vi "Path_2_String.vi"(1 "Real Path":path) -> (0 "Path String":string)   [LabVIEW 2022 SP3]
uses:
  Globals/Constants_global.vi
  Globals/Preference_global.vi
panel:
  in  "POSIXFormattedPseudopath (F)":bool
  out "Data Folder":path
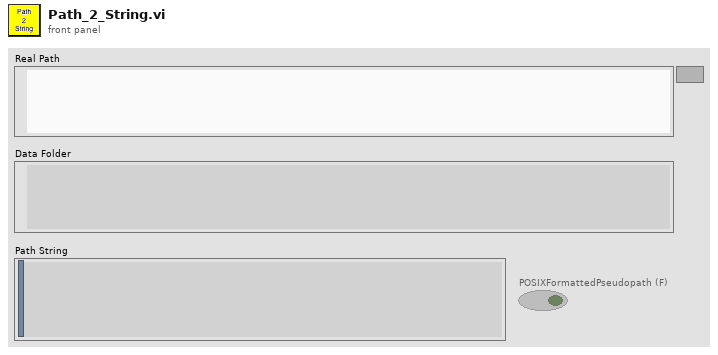
[diagram p1: front panel]
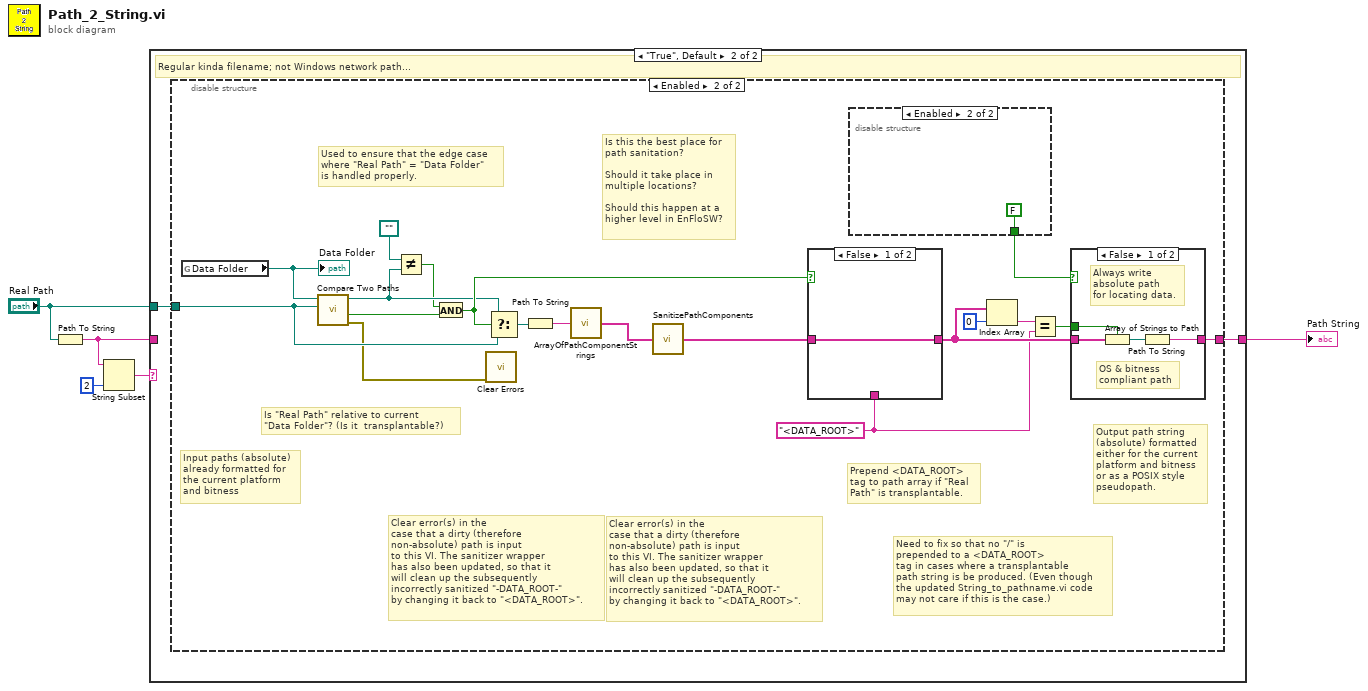
[diagram p0: block diagram]
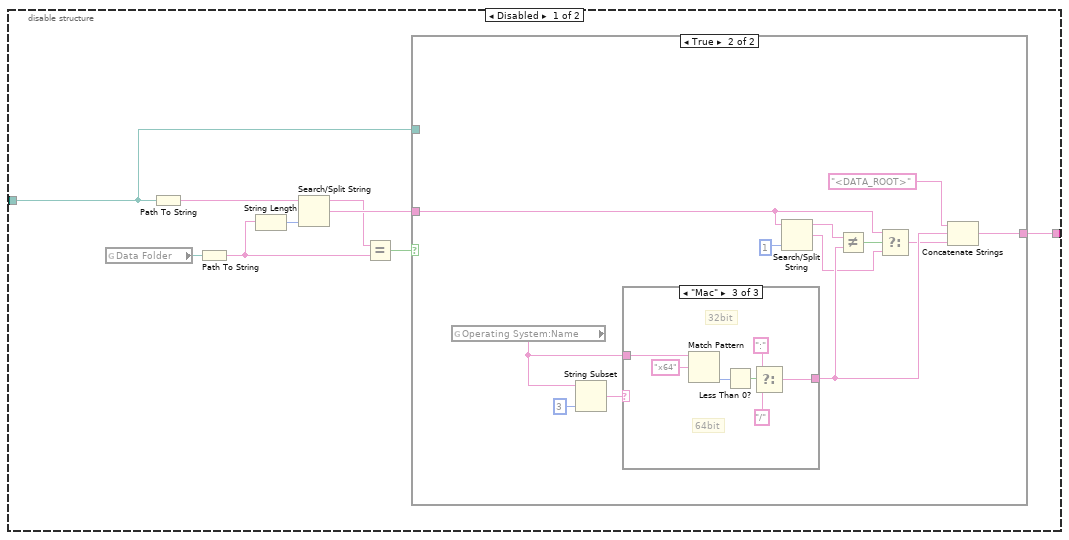
[diagram p3: hidden frame]
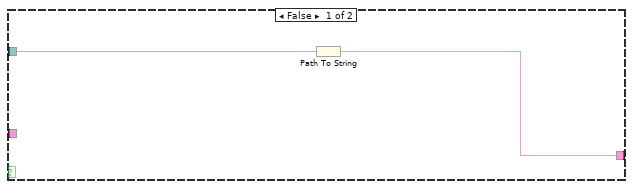
[diagram p4: hidden frame]
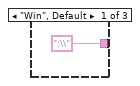
[diagram p5: hidden frame]
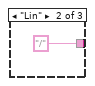
[diagram p6: hidden frame]
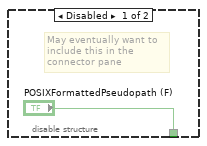
[diagram p7: hidden frame]
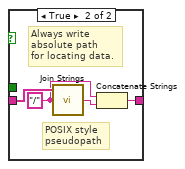
[diagram p8: hidden frame]
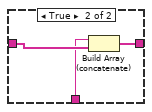
[diagram p9: hidden frame]
diagram:
  n1 = Path To String(path="Real Path") -> (string=w3:string)
  n2 = String Subset(string=w3, length (rest)=2 ("length (rest)")) -> (substring=w2:string)  [unwired: 1 in]
  n3 = case shown="\"True\", Default" w2 {
    tunnel: [w6 w8] -> w5
    tunnel: "Real Path" -> [_ w7]
    tunnel: w3 -> [w6 _]
    frame "\\\\" {
      # "String begins with \"\\\\\" (needs extra \\ for each \\ to match pattern!) meaning it is a Windows network path- just pass it, hope it's clean! (That's what used to happen!)"
    }
    frame "True", Default {
      # "Regular kinda filename; not Windows network path..."
      n4 = disable-structure shown="Enabled" {
        disable-tunnel: w7 -> [w10 w53]
        disable-tunnel: [w9 w52] -> w8
        frame Disabled {
          n5 = global read "Constants_global.vi" "Data Folder"() -> (w11:path)
          n6 = Path To String(path=w10) -> (string=w13:string)
          n7 = Path To String(path=w11) -> (string=w14:string)
          n8 = String Length(string=w14) -> (length=w12:i32)
          n9 = Search/Split String(string=w13, offset (0)=w12) -> (substring before match=w16:string, match + rest of string=w17:string)  [unwired: 1 in, 1 out]
          n10 = Equal?(x=w16, y=w14) -> (x = y?=w15:bool)
          n11 = case shown="True" w15 {
            tunnel: w10 -> [w19 _]
            tunnel: [w18 w30] -> w9
            tunnel: w17 -> [_ w21]
            frame False {
              n12 = Path To String(path=w19) -> (string=w18:string)
            }
            frame True {
              n13 = global read "Preference_global.vi" "Operating System:Name"() -> (w20:string)
              n14 = String Subset(string=w20, length (rest)=3 ("length (rest)")) -> (substring=w28:string)  [unwired: 1 out]
              n15 = case shown="\"Mac\"" w28 {
                tunnel: [":\\" "/" w35] -> w26
                tunnel: w20 -> [_ _ w40]
                frame "Win", Default {
                }
                frame "Lin" {
                }
                frame "Mac" {
                  # "64bit"
                  # "32bit"
                  n16 = Match Pattern(string=w40, regular expression="x64") -> (offset past match=w38:i32)  [unwired: 1 in, 3 out]
                  n17 = Less Than 0?(x=w38) -> (x < 0?=w37:bool)
                  n18 = Select(t=":", s=w37, f="/") -> (s? t:f=w35:string)
                }
              }
              n19 = Search/Split String(string=w21, offset (0)=1 ("length (rest)")) -> (substring before match=w23:string, match + rest of string=w24:string)  [unwired: 2 out]
              n20 = Not Equal?(x=w23, y=w26) -> (x != y?=w25:bool)
              n21 = Select(t=w21, s=w25, f=w24) -> (s? t:f=w22:string)
              n22 = Concatenate Strings("<DATA_ROOT>", w26, w22) -> (w30:string)
            }
          }
        }
        frame Enabled {
          w47 = "<DATA_ROOT>"
          # "Used to ensure that the edge case\nwhere \"Real Path\" = \"Data Folder\"\nis handled properly."
          # "Need to fix so that no \"/\" is\nprepended to a <DATA_ROOT>\ntag in cases where a transplantable\npath string is be produced. (Even though\nthe updated String_to_pathname.vi code\nmay not care if this is the case.)"
          # "Clear error(s) in the\ncase that a dirty (therefore\nnon-absolute) path is input\nto this VI. The sanitizer wrapper\nhas also been updated, so that it\nwill clean up the subsequently\nincorrectly sanitized \"-DATA_ROOT-\"\nby changing it back to \"<DATA_ROOT>\"."
          # "Clear error(s) in the\ncase that a dirty (therefore\nnon-absolute) path is input\nto this VI. The sanitizer wrapper\nhas also been updated, so that it\nwill clean up the subsequently\nincorrectly sanitized \"-DATA_ROOT-\"\nby changing it back to \"<DATA_ROOT>\"."
          # "Output path string\n(absolute) formatted\neither for the current\nplatform and bitness\nor as a POSIX style\npseudopath."
          # "Is this the best place for\npath sanitation?\n\nShould it take place in\nmultiple locations?\n\nShould this happen at a\nhigher level in EnFloSW?"
          # "Input paths (absolute)\nalready formatted for\nthe current platform \nand bitness"
          # "Is \"Real Path\" relative to current\n\"Data Folder\"? (Is it  transplantable?)"
          # "Prepend <DATA_ROOT>\ntag to path array if \"Real\nPath\" is transplantable."
          # "Input paths (absolute)\nalready formatted for\nthe current platform \nand bitness"
          n23 = global read "Constants_global.vi" "Data Folder"() -> (w54:path)
          "Data Folder" <- w54
          n24 = call <vilib>:"Compare Two Paths.vi"("Path 2"=w53, "Path 1"=w54) -> ("error out"=w51:errorcluster, "Path 2 Relative to Path 1?"=w44:bool, "Relative Path from 1 to 2"=w43:path)  [unwired: 6 in, 1 out]
          n25 = Not Equal?(x=path "", y=w43) -> (x != y?=w41:bool)
          n26 = And(x=w41, y=w44) -> (x .and. y?=w45:bool)
          n27 = call <vilib>:"Clear Errors.vi"("error in (no error)"=w51) -> ()  [unwired: 5 in, 2 out]
          n28 = Select(t=w43, s=w45, f=w53) -> (s? t:f=w55:path)
          n29 = Path To String(path=w55) -> (string=w57:string)
          n30 = call "ArrayOfPathComponentStrings.vi"("PathStringIn"=w57) -> ("ArrayOfPathComponentStringsOut"=w59:string[])
          n31 = call "SanitizePathComponents.vi"("PathComponentsIn"=w59) -> ("SanitizedComponentsOut"=w58:string[])
          n32 = case shown="False" w45 {
            tunnel: [w70 w73] -> w50
            tunnel: w58 -> [w70 w72]
            tunnel: w47 -> [_ w71]
            frame False {
            }
            frame True {
              n33 = Build Array (concatenate)(w71, w72) -> (w73:string[])
            }
          }
          n34 = disable-structure shown="Enabled" {
            disable-tunnel: ["POSIXFormattedPseudopath (F)" FALSE ("POSIXFormattedPseudopath (F)")] -> w56
            frame Disabled {
              # "May eventually want to\ninclude this in the\nconnector pane"
            }
            frame Enabled {
            }
          }
          n35 = Index Array(array=w50, index=0) -> (element=w48:string)
          n36 = Equal?(x=w48, y=w47) -> (x = y?=w46:bool)
          n37 = case shown="False" w56 {
            tunnel: w50 -> [w63 w69]
            tunnel: [w64 w68] -> w52
            tunnel: w46 -> [w62 _]
            frame False {
              # "OS & bitness\ncompliant path"
              # "Always write\nabsolute path\nfor locating data."
              n38 = Array of Strings to Path(0:w63, 1:w62) -> (2:w65:path)
              n39 = Path To String(path=w65) -> (string=w64:string)
            }
            frame True {
              w66 = "/" ("Separator (,)")
              # "POSIX style\npseudopath"
              # "Always write\nabsolute path\nfor locating data."
              n40 = call <vilib>:"Join Strings.vi"("Separator (,)"=w66, "Strings In"=w69) -> ("String"=w67:string)  [unwired: 1 in]
              n41 = Concatenate Strings(w66, w67) -> (w68:string)
            }
          }
        }
      }
    }
  }
  "Path String" <- w5
